vi "Update Mouse Enter.vi"(8 "error in (no error)":errorcluster, 11 "UI Controller in":refnum<class "UI Controller.lvclass">) -> (0 "error out":errorcluster, 3 "UI Controller out":refnum<class "UI Controller.lvclass">)   [LabVIEW 2020, in "UI Controller.lvlib" / "UI Controller.lvclass"]
uses:
  UI Controller.lvclass
  C:/Program Files/National Instruments/LabVIEW 2020/vi.lib/ActorFrameworkMVC/Abstract Controller/Abstract Controller/Abstract Controller.lvclass
  UI Controller.lvclass/UI Controller.ctl
  <vilib>/Utility/cursorutil.llb/Set Cursor (Cursor ID).vi
  <vilib>/ActorFrameworkMVC/Abstract Controller/Abstract Controller/Abstract Controller.lvclass
panel:
  # "NOTICE -- YOU MUST LEAVE THIS NOTICE IN PLACE.\n\nCopyright (c) 2017, LIANG LIU Shawn.Liu.cn@gmail.com\nAll rights reserved.\n\nRedistribution and use in source and binary forms, with or without modification, are permitted provided that the following conditions are met:\n-Redistributions of source code must retain the above copyright notice, this list of conditions and the following disclaimer.\n-Redistributions in binary form must reproduce the above copyright notice, this list of conditions and the following disclaimer in the documentation and/or other materials provided with the distribution.\n-Neither the name of the eLp nor the names of its contributors may be used to endorse or promote products derived from this software without specific prior written permission.\n\nTHIS SOFTWARE IS PROVIDED BY THE COPYRIGHT HOLDERS AND CONTRIBUTORS \"AS IS\" AND ANY EXPRESS OR IMPLIED WARRANTIES, INCLUDING, BUT NOT LIMITED TO, THE IMPLIED WARRANTIES OF MERCHANTABILITY AND FITNESS FOR A PARTICULAR PURPOSE ARE DISCLAIMED. IN NO EVENT SHALL THE COPYRIGHT HOLDER OR CONTRIBUTORS BE LIABLE FOR ANY DIRECT, INDIRECT, INCIDENTAL, SPECIAL, EXEMPLARY, OR CONSEQUENTIAL DAMAGES (INCLUDING, BUT NOT LIMITED TO, PROCUREMENT OF SUBSTITUTE GOODS OR SERVICES; LOSS OF USE, DATA, OR PROFITS; OR BUSINESS INTERRUPTION) HOWEVER CAUSED AND ON ANY THEORY OF LIABILITY, WHETHER IN CONTRACT, STRICT LIABILITY, OR TORT (INCLUDING NEGLIGENCE OR OTHERWISE) ARISING IN ANY WAY OUT OF THE USE OF THIS SOFTWARE, EVEN IF ADVISED OF THE POSSIBILITY OF SUCH DAMAGE."
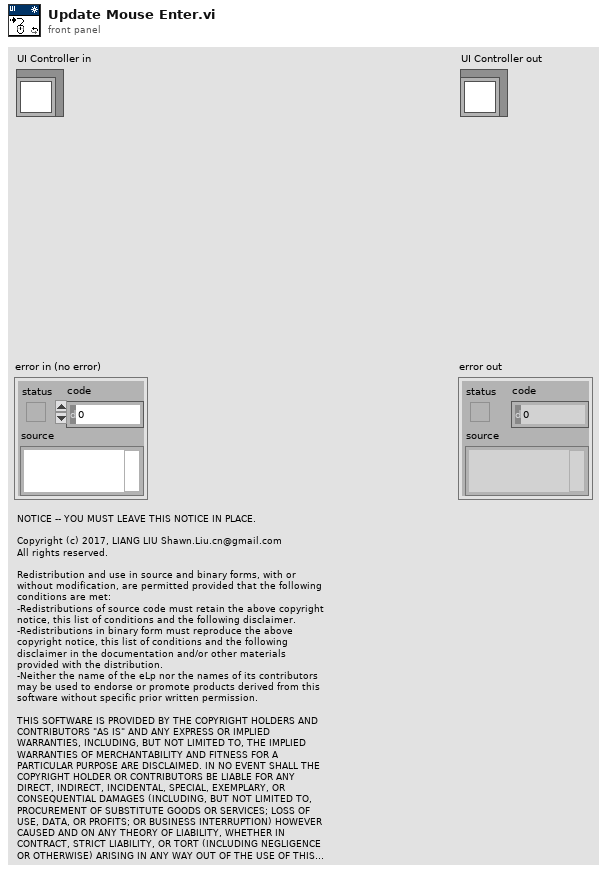
[diagram p1: front panel]
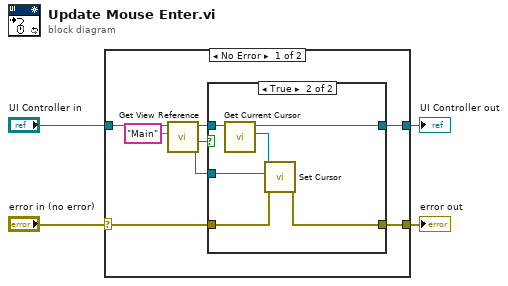
[diagram p0: block diagram]
diagram:
  n1 = case shown="No Error" "error in (no error)" {
    selector: "error in (no error)" -> [w6 w22]
    tunnel: "UI Controller in" -> [w12 w21]
    tunnel: [w11 w21] -> w3
    tunnel: [w5 w22] -> w1
    frame No Error {
      n2 = call <vilib>:"Get View Reference.vi"("View Name"="Main", "Abstract Controller in"=w12) -> ("Found?"=w8:bool, "VI Reference"=w7:refnum<vi>, "Abstract Controller out"=w9:refnum<class "UI Controller.lvclass">)  [unwired: 6 in, 1 out]
      n3 = case shown="True" w8 {
        tunnel: w9 -> [w14 w20]
        tunnel: w7 -> [_ w19]
        tunnel: [w14 w18] -> w11
        tunnel: w6 -> [w13 w16]
        tunnel: [w13 w15] -> w5
        frame False {
        }
        frame True {
          n4 = call "Get Current Cursor.vi"("UI Controller in"=w20) -> ("Current Cursor"=w17:refnum<k1>, "UI Controller out"=w18:refnum<class "UI Controller.lvclass">)  [unwired: 9 in]
          n5 = call-poly <vilib>:"Set Cursor.vi"("error in (no error)"=w16, "VI reference (current VI)"=w19, "cursor ID"=w17) -> ("error out"=w15:errorcluster)  [unwired: 7 in, 1 out]
        }
      }
    }
    frame Error {
    }
  }
  "error out" <- w1
  "UI Controller out" <- w3
